vi "UIM Values.vi"() -> ()   [LabVIEW 2020]
uses:
  UIM Class/UIM.lvclass
panel:
  in  "Boolean":bool=TRUE
  in  "Tab Control":enum32{"Cat", "Dog"}(tab)
  in  "File Path Control":path=path "c:/some_file.txt"
  in  "Horizontal Pointer Slide":dbl(slide)=2.222222 scale=0.0..10.0
  out "Meter":dbl(knob)=2.52 scale=0.0..10.0
  in  "Knob":dbl(knob)=3.0 scale=0.0..10.0
  in  "Menu Ring":u16(ring)=2 items=["I dont know", "Option 2", "Option 1"]
  in  "Enum":T1(ring)=enum."First Value"
  in  "String":string="Pi"
  in  "Numeric Control":dbl=3.14
  in  "Stop Button":bool
  in  "UI State":u16(ring) items=["Set1", "Set2", "default"]
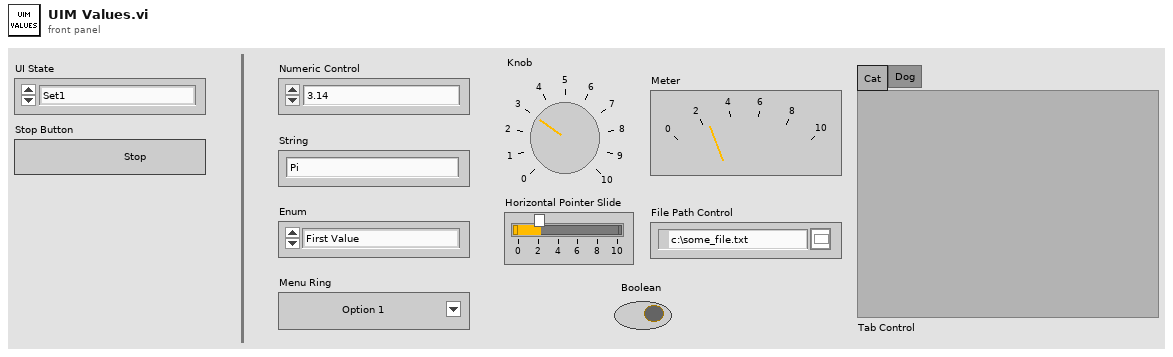
[diagram p1: front panel]
types:
  T1 = enum16{"Something Else", "Second Value", "First Value"}
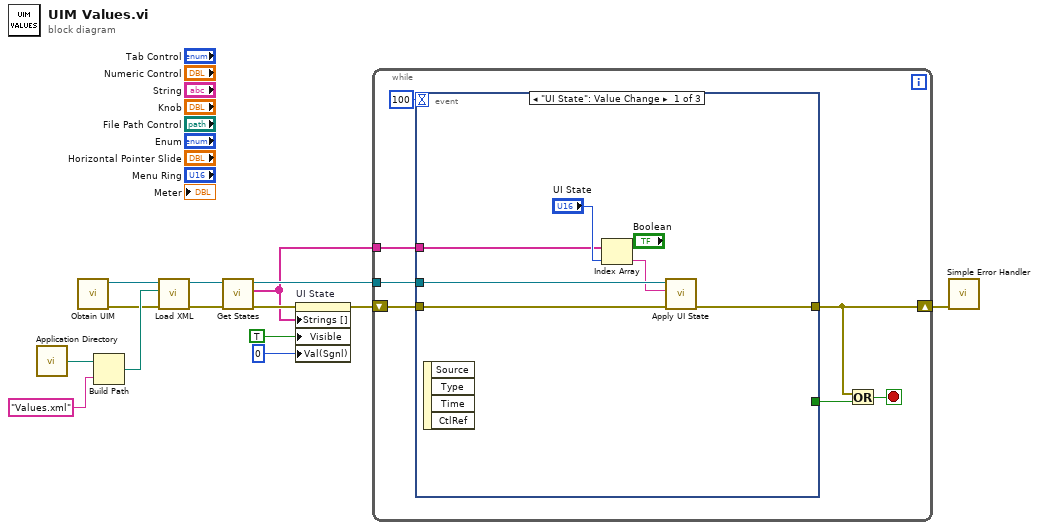
[diagram p0: block diagram]
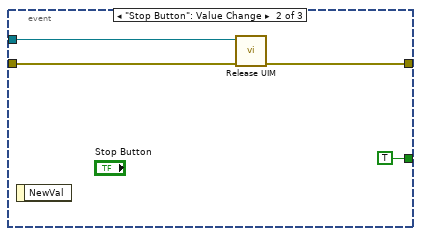
[diagram p2: hidden frame]
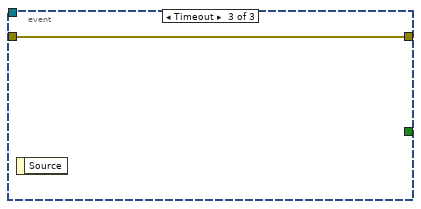
[diagram p3: hidden frame]
diagram:
  n1 = call <vilib>:"Application Directory.vi"() -> ("Application Directory"=w1:path)
  n2 = call "Obtain UIM.vi"() -> ("Error Out"=w4:errorcluster, "UIM Handle"=w11:refnum<data-value>)  [unwired: 10 in]
  n3 = Build Path(base path=w1, name or relative path="Values.xml") -> (appended path=w5:path)
  n4 = call "Load XML.vi"("Error In"=w4, "XML File"=w5, "UIM In"=w11) -> ("Error Out"=w7:errorcluster, "UIM Out"=w10:refnum<data-value>)  [unwired: 7 in]
  n5 = call "Get States.vi"("Error In"=w7, "UIM In"=w10) -> ("Error Out"=w8:errorcluster, "States"=w3:string[], "UIM Out"=w9:refnum<data-value>)  [unwired: 7 in]
  n6 = property on="UI State" class="Ring (strict)"(error in=w8, "Strings []"=w3, "Visible"=TRUE, "Val(Sgnl)"=u16 0 ("Value (Signaling)")) -> (error out=w14:errorcluster)  [unwired: 1 in, 1 out]
  n7 = while {
    tunnel: w9 -> [w21]
    tunnel: w3 -> [w19]
    shift-right: [w16] -> w2
    shift-left: w14 -> [w20]
    stop <- w17 stop-if-true
    n8 = event shown="[0] \"UI State\": Value Change" {
      selector: _ -> [_ _ _]
      dyn-events: _ -> [_ _ _]
      timeout: 100 -> [_ _ _]
      tunnel: w21 -> [w27 w30 _]
      tunnel: [_ TRUE _] -> w18
      tunnel: w20 -> [w26 w29 w32]
      tunnel: [w22 w28 w32] -> w16
      tunnel: w19 -> [w24 _ _]
      event "UI State": Value Change {
        n9 = event-data() -> ()  [unwired: 1 in, 4 out]
        n10 = Index Array(array=w24, index="UI State") -> (element=w23:string)
        n11 = call "Apply UI State.vi"("Error In"=w26, "State Name"=w23, "UIM In"=w27) -> ("Error Out"=w22:errorcluster)  [unwired: 7 in, 1 out]
      }
      event "Stop Button": Value Change {
        n12 = event-data() -> ()  [unwired: 1 in, 1 out]
        n13 = call "Release UIM.vi"("Error In"=w29, "UIM Handle"=w30) -> ("Error Out"=w28:errorcluster)  [unwired: 9 in]
      }
      event Timeout {
        n14 = event-data() -> ()  [unwired: 1 in, 1 out]
      }
    }
    n15 = Or(x=w16, y=w18) -> (x .or. y?=w17:bool)
  }
  n16 = call <vilib>:"Simple Error Handler.vi"("error in (no error)"=w2) -> ()  [unwired: 4 in, 5 out]
